vi "finalvi.vi"() -> ()   [LabVIEW 2022 SP3]
uses:
  <vilib>/MakerHub/LINX/Public/Peripherals/Analog/Analog Read 1 Chan.vi
  <vilib>/MakerHub/LINX/Public/Peripherals/Digital/Digital Write 1 Chan.vi
  <vilib>/MakerHub/LINX/Public/Peripherals/Analog/Analog Read N Chans.vi
  <vilib>/MakerHub/LINX/Public/Peripherals/Digital/Digital Write N Chans.vi
  <vilib>/MakerHub/LINX/Private/Local IO/LinxAnalogRead.vi
  <vilib>/MakerHub/LINX/Public/Utilities/Check Channel.vi
  <vilib>/MakerHub/LINX/Private/Local IO/LinxDigitalWrite.vi
  <vilib>/MakerHub/LINX/Public/Utilities/Open Serial.vi
  <vilib>/MakerHub/LINX/Private/Utilties/Generate Error.vi
  <vilib>/MakerHub/LINX/LMH-LINX.lvlib
panel:
  in  "DO Channel 101(13)":u8
  in  "DO Channel 102(12)":u8
  out "Value (0-100) 102":dbl
  in  "AI Channel 102":u8
  out "Value (0-100) 101":dbl
  in  "AI Channel 101":u8
  in  "DO Channel 201(11)":u8
  in  "DO Channel 202(10)":u8
  out "Value (0-100) 202":dbl
  in  "AI Channel 202":u8
  out "Value (0-100) 201":dbl
  in  "AI Channel 201":u8
  in  "DO Channel 301(9)":u8
  in  "DO Channel 302(8)":u8
  out "Value (0-100) 302":dbl
  in  "AI Channel 302":u8
  out "Value (0-100) 301":dbl
  in  "AI Channel 301":u8
  in  "VISA resource":refnum<visa-resource-name>
  in  "stop":bool
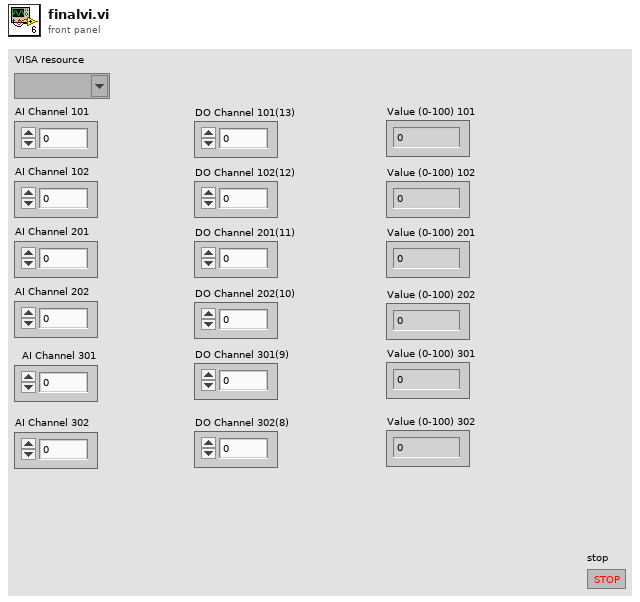
[diagram p1: front panel]
types:
  T1 = typedef "LMH-LINX.lvlib/LINX Ref.ctl" = cluster{"IO":T2, "Interface":T3, "LINX Device Config":T4}
  T2 = typedef "LMH-LINX.lvlib/Platform.ctl" = enum16{"Remote", "Local"}
  T3 = typedef "LMH-LINX.lvlib/Interface.ctl" = enum16{"Serial", "TCP"}
  T4 = typedef "LMH-LINX.lvlib/Device.lvlib/LINX Device Config.ctl" = cluster{"Interface":T3, "COM Port":refnum<visa-resource-name>, "TCP Configuration":T5, "Device Family":u8, "Device ID":u8, "Device Name":string, "TCP Ref":refnum<k5>, "Channels":T6}
  T5 = typedef "LMH-LINX.lvlib/Device.lvlib/TCP Config.ctl" = cluster{"IP Address":string, "Port":u16}
  T6 = typedef "LMH-LINX.lvlib/Channels.ctl" = cluster{"DI":u8[], "DO":u8[], "AI":u8[], "AO":u8[], "PWM":u8[], "QE":u8[], "UART":u8[], "I2C 2":u8[], "SPI":u8[], "CAN":u8[], "Servo":u8[], "AI Ref (V)":dbl, "AI Resolution (Bits)":u8, "AO Ref (V)":dbl, "AO Resolution (Bits)":u8}
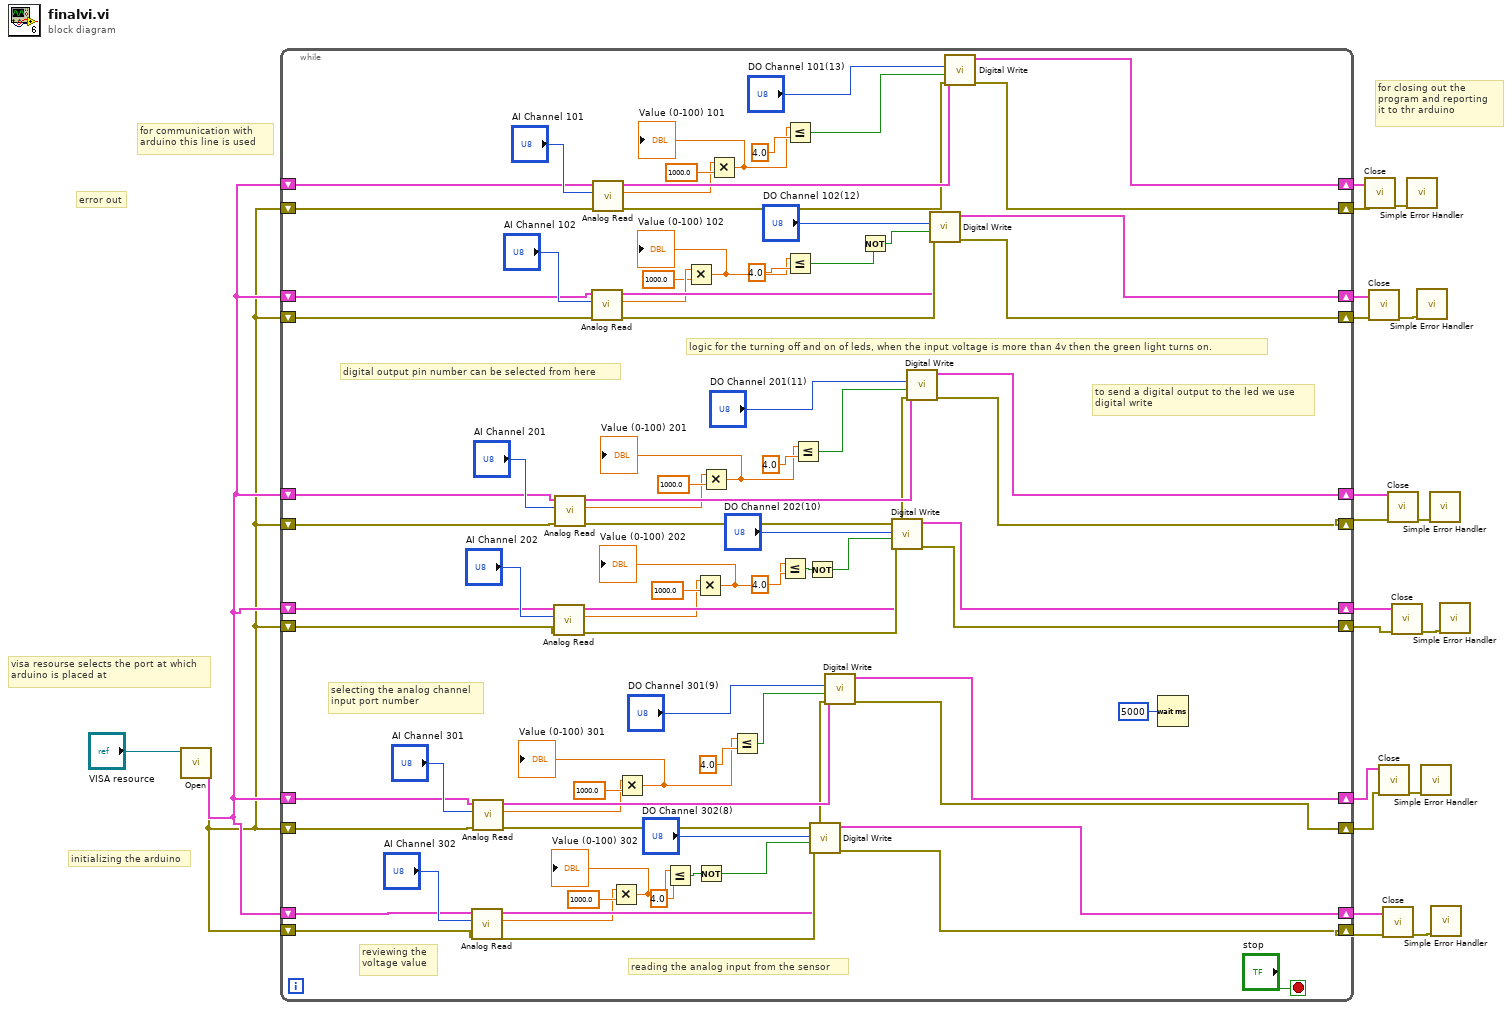
[diagram p0: block diagram]
diagram:
  # "error out"
  # "for communication with \narduino this line is used"
  # "for closing out the \nprogram and reporting \nit to thr arduino"
  # "initializing the arduino"
  # "visa resourse selects the port at which\narduino is placed at"
  n1 = call-poly <vilib>:"Open.vi"("Serial Port"="VISA resource") -> ("Error Out"=w7:errorcluster, "LINX Resource"=w8:T1)  [unwired: 8 in, 1 out]
  n2 = while {
    shift-right: [w87] -> w18
    shift-left: w8 -> [w88]
    shift-right: [w86] -> w17
    shift-left: w7 -> [w89]
    shift-right: [w85] -> w16
    shift-left: w8 -> [w91]
    shift-right: [w84] -> w15
    shift-left: w7 -> [w90]
    shift-right: [w68] -> w10
    shift-left: w8 -> [w72]
    shift-right: [w67] -> w9
    shift-left: w7 -> [w70]
    shift-right: [w66] -> w12
    shift-left: w8 -> [w71]
    shift-right: [w65] -> w11
    shift-left: w7 -> [w69]
    shift-right: [w48] -> w4
    shift-left: w8 -> [w52]
    shift-right: [w47] -> w3
    shift-left: w7 -> [w50]
    shift-right: [w46] -> w2
    shift-left: w8 -> [w51]
    shift-right: [w45] -> w1
    shift-left: w7 -> [w49]
    stop <- "stop" stop-if-true
    # "logic for the turning off and on of leds, when the input voltage is more than 4v then the green light turns on."
    # "digital output pin number can be selected from here"
    # "to send a digital output to the led we use \ndigital write"
    # "reviewing the \nvoltage value"
    # "reading the analog input from the sensor"
    # "selecting the analog channel\ninput port number"
    n3 = call-poly <vilib>:"Analog Read.vi"("Error In"=w89, "Analog Channel"="AI Channel 302", "LINX Resource"=w88) -> ("Error Out"=w97:errorcluster, "Voltage"=w37:dbl, "LINX Resource"=w96:T1)  [unwired: 5 in, 1 out]
    n4 = call-poly <vilib>:"Analog Read.vi"("Error In"=w90, "Analog Channel"="AI Channel 301", "LINX Resource"=w91) -> ("Error Out"=w24:errorcluster, "Voltage"=w34:dbl, "LINX Resource"=w100:T1)  [unwired: 5 in, 1 out]
    n5 = call-poly <vilib>:"Analog Read.vi"("Error In"=w69, "Analog Channel"="AI Channel 202", "LINX Resource"=w71) -> ("Error Out"=w78:errorcluster, "Voltage"=w30:dbl, "LINX Resource"=w77:T1)  [unwired: 5 in, 1 out]
    n6 = call-poly <vilib>:"Analog Read.vi"("Error In"=w70, "Analog Channel"="AI Channel 201", "LINX Resource"=w72) -> ("Error Out"=w25:errorcluster, "Voltage"=w27:dbl, "LINX Resource"=w80:T1)  [unwired: 5 in, 1 out]
    n7 = call-poly <vilib>:"Analog Read.vi"("Error In"=w49, "Analog Channel"="AI Channel 102", "LINX Resource"=w51) -> ("Error Out"=w58:errorcluster, "Voltage"=w44:dbl, "LINX Resource"=w57:T1)  [unwired: 5 in, 1 out]
    n8 = call-poly <vilib>:"Analog Read.vi"("Error In"=w50, "Analog Channel"="AI Channel 101", "LINX Resource"=w52) -> ("Error Out"=w23:errorcluster, "Voltage"=w41:dbl, "LINX Resource"=w61:T1)  [unwired: 5 in, 1 out]
    n9 = Multiply(x=w37, y=1000.0) -> (x*y=w35:dbl)
    "Value (0-100) 302" <- w35
    n10 = Multiply(x=w34, y=1000.0) -> (x*y=w33:dbl)
    "Value (0-100) 301" <- w33
    n11 = Less Or Equal?(x=w35, y=4.0) -> (x <= y?=w95:bool)
    n12 = Multiply(x=w44, y=1000.0) -> (x*y=w39:dbl)
    "Value (0-100) 102" <- w39
    n13 = Multiply(x=w30, y=1000.0) -> (x*y=w29:dbl)
    "Value (0-100) 202" <- w29
    n14 = Not(x=w95) -> (.not. x?=w94:bool)
    n15 = Multiply(x=w27, y=1000.0) -> (x*y=w26:dbl)
    "Value (0-100) 201" <- w26
    n16 = Multiply(x=w41, y=1000.0) -> (x*y=w40:dbl)
    "Value (0-100) 101" <- w40
    n17 = Less Or Equal?(x=w33, y=4.0) -> (x <= y?=w101:bool)
    n18 = Less Or Equal?(x=w29, y=4.0) -> (x <= y?=w76:bool)
    n19 = Less Or Equal?(x=w40, y=4.0) -> (x <= y?=w62:bool)
    n20 = Less Or Equal?(x=w39, y=4.0) -> (x <= y?=w56:bool)
    n21 = Less Or Equal?(x=w26, y=4.0) -> (x <= y?=w81:bool)
    n22 = Not(x=w76) -> (.not. x?=w75:bool)
    n23 = call-poly <vilib>:"Digital Write.vi"("Error In"=w97, "Output Value"=w94, "DO Channel"="DO Channel 302(8)", "LINX Resource"=w96) -> ("Error Out"=w86:errorcluster, "LINX Resource"=w87:T1)  [unwired: 6 in]
    n24 = call-poly <vilib>:"Digital Write.vi"("Error In"=w24, "Output Value"=w101, "DO Channel"="DO Channel 301(9)", "LINX Resource"=w100) -> ("Error Out"=w84:errorcluster, "LINX Resource"=w85:T1)  [unwired: 6 in]
    n25 = Not(x=w56) -> (.not. x?=w55:bool)
    n26 = call-poly <vilib>:"Digital Write.vi"("Error In"=w78, "Output Value"=w75, "DO Channel"="DO Channel 202(10)", "LINX Resource"=w77) -> ("Error Out"=w65:errorcluster, "LINX Resource"=w66:T1)  [unwired: 6 in]
    n27 = call-poly <vilib>:"Digital Write.vi"("Error In"=w25, "Output Value"=w81, "DO Channel"="DO Channel 201(11)", "LINX Resource"=w80) -> ("Error Out"=w67:errorcluster, "LINX Resource"=w68:T1)  [unwired: 6 in]
    n28 = call-poly <vilib>:"Digital Write.vi"("Error In"=w58, "Output Value"=w55, "DO Channel"="DO Channel 102(12)", "LINX Resource"=w57) -> ("Error Out"=w45:errorcluster, "LINX Resource"=w46:T1)  [unwired: 6 in]
    n29 = call-poly <vilib>:"Digital Write.vi"("Error In"=w23, "Output Value"=w62, "DO Channel"="DO Channel 101(13)", "LINX Resource"=w61) -> ("Error Out"=w47:errorcluster, "LINX Resource"=w48:T1)  [unwired: 6 in]
    n30 = Wait (ms)(milliseconds to wait=u32 5000) -> ()  [unwired: 1 out]
  }
  n31 = call <vilib>:"Close.vi"("Error In"=w3, "LINX Resource"=w4) -> ("Error Out"=w6:errorcluster)  [unwired: 9 in]
  n32 = call <vilib>:"Close.vi"("Error In"=w1, "LINX Resource"=w2) -> ("Error Out"=w5:errorcluster)  [unwired: 9 in]
  n33 = call <vilib>:"Close.vi"("Error In"=w15, "LINX Resource"=w16) -> ("Error Out"=w20:errorcluster)  [unwired: 9 in]
  n34 = call <vilib>:"Close.vi"("Error In"=w17, "LINX Resource"=w18) -> ("Error Out"=w19:errorcluster)  [unwired: 9 in]
  n35 = call <vilib>:"Close.vi"("Error In"=w9, "LINX Resource"=w10) -> ("Error Out"=w14:errorcluster)  [unwired: 9 in]
  n36 = call <vilib>:"Close.vi"("Error In"=w11, "LINX Resource"=w12) -> ("Error Out"=w13:errorcluster)  [unwired: 9 in]
  n37 = call <vilib>:"Simple Error Handler.vi"("error in (no error)"=w6) -> ()  [unwired: 4 in, 5 out]
  n38 = call <vilib>:"Simple Error Handler.vi"("error in (no error)"=w5) -> ()  [unwired: 4 in, 5 out]
  n39 = call <vilib>:"Simple Error Handler.vi"("error in (no error)"=w20) -> ()  [unwired: 4 in, 5 out]
  n40 = call <vilib>:"Simple Error Handler.vi"("error in (no error)"=w14) -> ()  [unwired: 4 in, 5 out]
  n41 = call <vilib>:"Simple Error Handler.vi"("error in (no error)"=w19) -> ()  [unwired: 4 in, 5 out]
  n42 = call <vilib>:"Simple Error Handler.vi"("error in (no error)"=w13) -> ()  [unwired: 4 in, 5 out]
